vi "Switch Application Mode.vi"(0 "VISA resource name":refnum<visa-resource-name>, 5 "Application Window (0:Active)":i32(ring) items=["Active", "Inactive", "Minimized", "Non", "Initialize"], 7 "Application Name (1:Spectrum Analyzer)":i32(ring)=1 items=["Signal Analyzer", "Spectrum Analyzer", "Phase Noise", "Config", "Signal Generator", "BER Test", "WiMAX", "W-CDMA/HSPA Downlink", "W-CDMA/HSPA Uplink", "GSM", "ETC/DSRC", "TD-SCDMA", "XG-PHS", "Vector Modulation Analysis", "3GLTE Downlink", "3GLTE Uplink", "LTE-TDD Downlink", "CDMA2000", "EVDO", "W-CDMA BS", "W-CDMA RNC Simulator Control", "MediaFLO", "ISDB-Tmm", "UMTS Measurement Software", "Digital I/F Control Software", "PA Measurement", "Power Meter"], 11 "error in (no error)":errorcluster) -> (4 "VISA resource name out":refnum<visa-resource-name>, 15 "error out":errorcluster)   [LabVIEW 2020, in "Anritsu Signal Analyzer Series.lvlib"]
doc: "Switches the target application for operation/control."
uses:
  Anritsu Signal Analyzer Series.lvlib
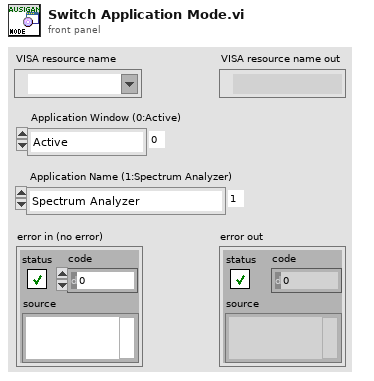
[diagram p1: front panel]
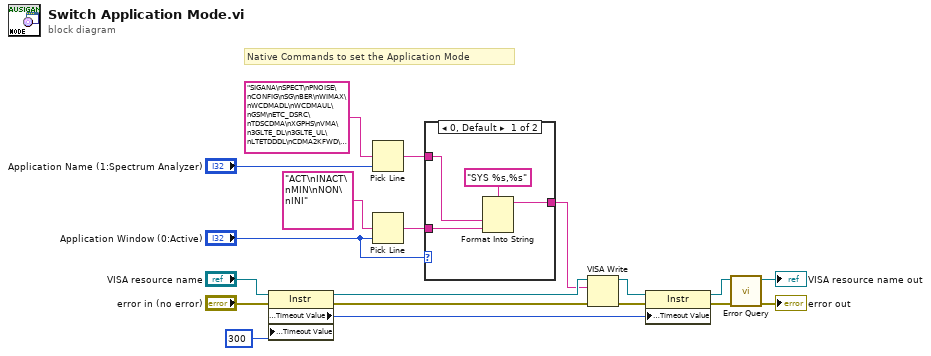
[diagram p0: block diagram]
diagram:
  # "Native Commands to set the Application Mode"
  n1 = property class="Instr"(reference="VISA resource name", error in="error in (no error)", "General Settings:Timeout Value"=u32 300) -> (reference out=w14:refnum<visa-resource-name>, error out=w13:errorcluster, "General Settings:Timeout Value"=w9:u32)
  n2 = Pick Line(multi-line string="SIGANA\nSPECT\nPNOISE\nCONFIG\nSG\nBER\nWIMAX\nWCDMADL\nWCDMAUL\nGSM\nETC_DSRC\nTDSCDMA\nXGPHS\nVMA\n3GLTE_DL\n3GLTE_UL\nLTETDDDL\nCDMA2KFWD\nEVDOFWD\nWCDMA_BS\nRNC\nMEDIAFLO\nISDBTMM\nUMTS\nBBIF\nPA\nPMET" ("文字列"), line index="Application Name (1:Spectrum Analyzer)") -> (output string=w5:string)  [unwired: 1 in]
  n3 = Pick Line(multi-line string="ACT\nINACT\nMIN\nNON\nINI" ("文字列"), line index="Application Window (0:Active)") -> (output string=w3:string)  [unwired: 1 in]
  n4 = case shown="0, Default" "Application Window (0:Active)" {
    tunnel: [w22 w24] -> w12
    tunnel: w5 -> [w21 _]
    tunnel: w3 -> [w20 w24]
    frame 0, Default {
      n5 = Format Into String(format string="SYS %s,%s" ("_Command Set"), w21, w20) -> (resulting string=w22:string)  [unwired: 2 in, 1 out]
    }
    frame 4 {
    }
  }
  n6 = VISA Write(VISA resource name=w14, write buffer=w12, error in (no error)=w13) -> (VISA resource name out=w11:refnum<visa-resource-name>, error out=w10:errorcluster)  [unwired: 1 out]
  n7 = property class="Instr"(reference=w11, error in=w10, "General Settings:Timeout Value"=w9) -> (reference out=w8:refnum<visa-resource-name>, error out=w7:errorcluster)
  n8 = call "Error Query.vi"("error in (no error)"=w7, "VISA resource name"=w8) -> ("error out"=→"error out":errorcluster, "VISA resource name out"=→"VISA resource name out":refnum<visa-resource-name>)  [unwired: 6 in, 2 out]
